vi "NMLDAQ_data_import.vi"(0 "NML Data Acquisition VI":string(combo)="NML Data Acquisition-New.vi") -> (1 "data":dbl[][](array[numeric])=[[0.0, 0.0], [0.481, 0.481], [0.98, 0.98], [1.48, 1.48], [1.98, 1.98], [2.48, 2.48], [2.98, 2.98], [3.48, 3.48], [3.98, 3.98], [4.48, 4.48], [4.98, 4.98], [5.48, 5.48], [5.98, 5.98], [6.48, 6.48], [6.98, 6.98], [7.48, 7.48], [7.98, 7.98], [8.48, 8.48], [8.98, 8.98], [9.48, 9.48], [9.98, 9.98], [10.48, 10.48], [10.98, 10.98], [11.48, 11.48], [11.981, 11.981], [12.48, 12.48], [12.981, 12.981], [13.48, 13.48], [13.98, 13.98], [14.48, 14.48], [14.98, 14.98], [15.48, 15.48], [15.981, 15.981], [16.48, 16.48], [16.981, 16.981], [17.48, 17.48], [17.98, 17.98], [18.48, 18.48], [18.981, 18.981], [19.48, 19.48], [19.98, 19.98], [20.48, 20.48], [20.981, 20.981], [21.48, 21.48], [21.981, 21.981], [22.48, 22.48], [22.981, 22.981], [23.48, 23.48], [23.981, 23.981], [24.48, 24.48], [24.981, 24.981], [25.48, 25.48], [25.98, 25.98], [26.48, 26.48], [26.981, 26.981], [27.48, 27.48], [27.981, 27.981], [28.48, 28.48], [28.981, 28.981], [29.48, 29.48], [29.981, 29.981], [30.48, 30.48], [30.981, 30.981], [31.48, 31.48], [31.98, 31.98], [32.48, 32.48], [32.98, 32.98], [33.48, 33.48], [33.98, 33.98], [34.48, 34.48], [34.98, 34.98], [35.48, 35.48], [35.98, 35.98], [36.48, 36.48], [36.98, 36.98], [37.48, 37.48], [37.98, 37.98], [38.48, 38.48], [38.98, 38.98], [39.48, 39.48], [39.98, 39.98], [40.48, 40.48], [40.98, 40.98], [41.48, 41.48], [41.98, 41.98], [42.48, 42.48], [42.98, 42.98], [43.48, 43.48], [43.98, 43.98], [44.48, 44.48], [44.98, 44.98], [45.48, 45.48], [45.98, 45.98], [46.481, 46.481], [46.98, 46.98], [47.48, 47.48], [47.98, 47.98], [48.48, 48.48], [48.98, 48.98], [49.48, 49.48], [49.98, 49.98], [50.48, 50.48], [50.98, 50.98], [51.48, 51.48], [51.981, 51.981], [52.48, 52.48], [52.981, 52.981], [53.48, 53.48], [53.981, 53.981], [54.48, 54.48], [54.981, 54.981], [55.48, 55.48], [55.981, 55.981], [56.481, 56.481], [56.98, 56.98], [57.48, 57.48], [57.98, 57.98], [58.48, 58.48], [58.98, 58.98], [59.48, 59.48], [59.98, 59.98], [60.48, 60.48], [60.98, 60.98], [61.48, 61.48], [61.98, 61.98], [62.48, 62.48], [62.98, 62.98], [63.48, 63.48], [63.98, 63.98], [64.48, 64.48], [64.98, 64.98], [65.48, 65.48], [65.98, 65.98], [66.481, 66.481], [66.98, 66.98], [67.48, 67.48], [67.98, 67.98], [68.48, 68.48], [68.98, 68.98], [69.48, 69.48], [69.98, 69.98], [70.48, 70.48], [70.98, 70.98], [71.48, 71.48], [71.981, 71.981], [72.48, 72.48], [72.98, 72.98], [73.48, 73.48], [73.98, 73.98], [74.48, 74.48], [74.98, 74.98], [75.48, 75.48], [75.98, 75.98], [76.48, 76.48], [76.98, 76.98], [77.48, 77.48], [77.981, 77.981], [78.48, 78.48], [78.981, 78.981], [79.48, 79.48], [79.981, 79.981], [80.48, 80.48], [80.981, 80.981], [81.48, 81.48], [81.981, 81.981], [82.48, 82.48], [82.981, 82.981], [83.48, 83.48], [83.981, 83.981], [84.48, 84.48], [84.981, 84.981], [85.48, 85.48], [85.981, 85.981], [86.48, 86.48], [86.98, 86.98], [87.48, 87.48], [87.981, 87.981], [88.48, 88.48], [88.981, 88.981], [89.48, 89.48], [89.98, 89.98], [90.48, 90.48], [90.98, 90.98], [91.48, 91.48], [91.98, 91.98], [92.48, 92.48], [92.98, 92.98], [93.48, 93.48], [93.98, 93.98], [94.48, 94.48], [94.98, 94.98], [95.48, 95.48], [95.981, 95.981], [96.48, 96.48], [96.98, 96.98], [97.48, 97.48], [97.98, 97.98], [98.48, 98.48], [98.981, 98.981], [99.48, 99.48], [99.981, 99.981], [100.48, 100.48], [100.98, 100.98], [101.48, 101.48], [101.981, 101.981], [102.48, 102.48], [102.981, 102.981], [103.48, 103.48], [103.981, 103.981], [104.48, 104.48], [104.98, 104.98], [105.48, 105.48], [105.98, 105.98], [106.48, 106.48], [106.981, 106.981], [107.48, 107.48], [107.981, 107.981], [108.48, 108.48], [108.981, 108.981], [109.48, 109.48], [109.981, 109.981], [110.48, 110.48], [110.981, 110.981], [111.48, 111.48], [111.981, 111.981], [112.48, 112.48], [112.981, 112.981], [113.48, 113.48], [113.981, 113.981], [114.48, 114.48], [114.981, 114.981], [115.48, 115.48], [115.981, 115.981], [116.48, 116.48], [116.981, 116.981], [117.48, 117.48], [117.981, 117.981], [118.48, 118.48], [118.981, 118.981], [119.48, 119.48], [119.981, 119.981], [120.48, 120.48], [120.981, 120.981], [121.48, 121.48], [121.981, 121.981], [122.48, 122.48], [122.981, 122.981], [123.48, 123.48], [123.981, 123.981], [124.48, 124.48], [124.981, 124.981], [125.48, 125.48], [125.981, 125.981], [126.48, 126.48], [126.981, 126.981], [127.48, 127.48], [127.981, 127.981], [128.48, 128.48], [128.981, 128.981], [129.48, 129.48], [129.981, 129.981], [130.48, 130.48], [130.981, 130.981], [131.48, 131.48], [131.981, 131.981], [132.48, 132.48], [132.981, 132.981], [133.48, 133.48], [133.981, 133.981], [134.48, 134.48], [134.981, 134.981], [135.48, 135.48], [135.981, 135.981], [136.48, 136.48], [136.981, 136.981], [137.48, 137.48], [137.981, 137.981], [138.48, 138.48], [138.981, 138.981], [139.48, 139.48], [139.981, 139.981], [140.48, 140.48], [140.981, 140.981], [141.48, 141.48], [141.981, 141.981], [142.48, 142.48], [142.981, 142.981], [143.48, 143.48], [143.981, 143.981], [144.48, 144.48], [144.981, 144.981], [145.48, 145.48], [145.981, 145.981], [146.48, 146.48], [146.981, 146.981], [147.48, 147.48], [147.981, 147.981], [148.48, 148.48], [148.981, 148.981], [149.48, 149.48], [149.981, 149.981], [150.48, 150.48], [150.981, 150.981], [151.48, 151.48], [151.981, 151.981], [152.48, 152.48], [152.98, 152.98], [153.48, 153.48], [153.981, 153.981], [154.48, 154.48], [154.981, 154.981], [155.48, 155.48], [155.981, 155.981], [156.48, 156.48], [156.981, 156.981], [157.48, 157.48], [157.98, 157.98], [158.48, 158.48], [158.981, 158.981], [159.48, 159.48], [159.98, 159.98], [160.48, 160.48], [160.981, 160.981], [161.48, 161.48], [161.981, 161.981], [162.48, 162.48], [162.98, 162.98], [163.48, 163.48], [163.98, 163.98], [164.48, 164.48], [164.98, 164.98], [165.48, 165.48], [165.981, 165.981], [166.48, 166.48], [166.981, 166.981], [167.48, 167.48], [167.981, 167.981], [168.48, 168.48], [168.98, 168.98], [169.48, 169.48], [169.981, 169.981], [170.48, 170.48], [170.981, 170.981], [171.48, 171.48], [171.981, 171.981], [172.48, 172.48], [172.98, 172.98], [173.48, 173.48], [173.98, 173.98], [174.48, 174.48], [174.981, 174.981], [175.48, 175.48], [nan, nan], [nan, nan], [nan, nan], [nan, nan], [nan, nan], [nan, nan], [nan, nan], [nan, nan], [nan, nan], [nan, nan], [nan, nan], [nan, nan], [nan, nan], [nan, nan], [nan, nan], [nan, nan], [nan, nan], [nan, nan], [nan, nan], [nan, nan], [nan, nan], [nan, nan], [nan, nan], [nan, nan], [nan, nan], [nan, nan], [nan, nan], [nan, nan], [nan, nan], [nan, nan], [nan, nan], [nan, nan], [nan, nan], [nan, nan], [nan, nan], [nan, nan], [nan, nan], [nan, nan], [nan, nan], [nan, nan], [nan, nan], [nan, nan], [nan, nan], [nan, nan], [nan, nan], [nan, nan], [nan, nan], [nan, nan], [nan, nan], [nan, nan], [nan, nan], [nan, nan], [nan, nan], [nan, nan], [nan, nan], [nan, nan], [nan, nan], [nan, nan], [nan, nan], [nan, nan], [nan, nan], [nan, nan], [nan, nan], [nan, nan], [nan, nan], [nan, nan], [nan, nan], [nan, nan], [nan, nan], [nan, nan], [nan, nan], [nan, nan], [nan, nan], [nan, nan], [nan, nan], [nan, nan], [nan, nan], [nan, nan], [nan, nan], [nan, nan], [nan, nan], [nan, nan], [nan, nan], [nan, nan], [nan, nan], [nan, nan], [nan, nan], [nan, nan], [nan, nan], [nan, nan], [nan, nan], [nan, nan], [nan, nan], [nan, nan], [nan, nan], [nan, nan], [nan, nan], [nan, nan], [nan, nan], [nan, nan], [nan, nan], [nan, nan], [nan, nan], [nan, nan], [nan, nan], [nan, nan], [nan, nan], [nan, nan], [nan, nan], [nan, nan], [nan, nan], [nan, nan], [nan, nan], [nan, nan], [nan, nan], [nan, nan], [nan, nan], [nan, nan], [nan, nan], [nan, nan], [nan, nan], [nan, nan], [nan, nan], [nan, nan], [nan, nan], [nan, nan], [nan, nan], [nan, nan], [nan, nan], [nan, nan], [nan, nan], [nan, nan], [nan, nan], [nan, nan], [nan, nan], [nan, nan], [nan, nan], [nan, nan], [nan, nan], [nan, nan], [nan, nan], [nan, nan], [nan, nan], [nan, nan], [nan, nan], [nan, nan], [nan, nan], [nan, nan], [nan, nan], [nan, nan], [nan, nan], [nan, nan], [nan, nan], [nan, nan], [nan, nan], [nan, nan], [nan, nan], [nan, nan], [nan, nan], [nan, nan], [nan, nan], [nan, nan], [nan, nan], [nan, nan], [nan, nan], [nan, nan], [nan, nan], [nan, nan], [nan, nan], [nan, nan], [nan, nan], [nan, nan], [nan, nan], [nan, nan], [nan, nan], [nan, nan], [nan, nan], [nan, nan], [nan, nan], [nan, nan], [nan, nan], [nan, nan], [nan, nan], [nan, nan], [nan, nan], [nan, nan], [nan, nan], [nan, nan], [nan, nan], [nan, nan], [nan, nan], [nan, nan], [nan, nan], [nan, nan], [nan, nan], [nan, nan], [nan, nan], [nan, nan], [nan, nan], [nan, nan], [nan, nan], [nan, nan], [nan, nan], [nan, nan], [nan, nan], [nan, nan], [nan, nan], [nan, nan], [nan, nan], [nan, nan], [nan, nan], [nan, nan], [nan, nan], [nan, nan], [nan, nan], [nan, nan], [nan, nan], [nan, nan], [nan, nan], [nan, nan], [nan, nan], [nan, nan], [nan, nan], [nan, nan], [nan, nan], [nan, nan], [nan, nan], [nan, nan], [nan, nan], [nan, nan], [nan, nan], [nan, nan], [nan, nan], [nan, nan], [nan, nan], [nan, nan], [nan, nan], [nan, nan], [nan, nan], [nan, nan], [nan, nan], [nan, nan], [nan, nan], [nan, nan], [nan, nan], [nan, nan], [nan, nan], [nan, nan], [nan, nan], [nan, nan], [nan, nan], [nan, nan], [nan, nan], [nan, nan], [nan, nan], [nan, nan], [nan, nan], [nan, nan], [nan, nan], [nan, nan], [nan, nan], [nan, nan], [nan, nan], [nan, nan], [nan, nan], [nan, nan], [nan, nan], [nan, nan], [nan, nan], [nan, nan], [nan, nan], [nan, nan], [nan, nan], [nan, nan], [nan, nan], [nan, nan], [nan, nan], [nan, nan], [nan, nan], [nan, nan], [nan, nan], [nan, nan], [nan, nan], [nan, nan], [nan, nan], [nan, nan], [nan, nan], [nan, nan], [nan, nan], [nan, nan], [nan, nan], [nan, nan], [nan, nan], [nan, nan], [nan, nan], [nan, nan], [nan, nan], [nan, nan], [nan, nan], [nan, nan], [nan, nan], [nan, nan], [nan, nan], [nan, nan], [nan, nan], [nan, nan], [nan, nan], [nan, nan], [nan, nan], [nan, nan], [nan, nan], [nan, nan], [nan, nan], [nan, nan], [nan, nan], [nan, nan], [nan, nan], [nan, nan], [nan, nan], [nan, nan], [nan, nan], [nan, nan], [nan, nan], [nan, nan], [nan, nan], [nan, nan], [nan, nan], [nan, nan], [nan, nan], [nan, nan], [nan, nan], [nan, nan], [nan, nan], [nan, nan], [nan, nan], [nan, nan], [nan, nan], [nan, nan], [nan, nan], [nan, nan], [nan, nan], [nan, nan], [nan, nan], [nan, nan], [nan, nan], [nan, nan], [nan, nan], [nan, nan], [nan, nan], [nan, nan], [nan, nan], [nan, nan], [nan, nan], [nan, nan], [nan, nan], [nan, nan], [nan, nan], [nan, nan], [nan, nan], [nan, nan], [nan, nan], [nan, nan], [nan, nan], [nan, nan], [nan, nan], [nan, nan], [nan, nan], [nan, nan], [nan, nan], [nan, nan], [nan, nan], [nan, nan], [nan, nan], [nan, nan], [nan, nan], [nan, nan], [nan, nan], [nan, nan], [nan, nan], [nan, nan], [nan, nan], [nan, nan], [nan, nan], [nan, nan], [nan, nan], [nan, nan], [nan, nan], [nan, nan], [nan, nan], [nan, nan], [nan, nan], [nan, nan], [nan, nan], [nan, nan], [nan, nan], [nan, nan], [nan, nan], [nan, nan], [nan, nan], [nan, nan], [nan, nan], [nan, nan], [nan, nan], [nan, nan], [nan, nan], [nan, nan], [nan, nan], [nan, nan], [nan, nan], [nan, nan], [nan, nan], [nan, nan], [nan, nan], [nan, nan], [nan, nan], [nan, nan], [nan, nan], [nan, nan], [nan, nan], [nan, nan], [nan, nan], [nan, nan], [nan, nan], [nan, nan], [nan, nan], [nan, nan], [nan, nan], [nan, nan], [nan, nan], [nan, nan], [nan, nan], [nan, nan], [nan, nan], [nan, nan], [nan, nan], [nan, nan], [nan, nan], [nan, nan], [nan, nan], [nan, nan], [nan, nan], [nan, nan], [nan, nan], [nan, nan], [nan, nan], [nan, nan], [nan, nan], [nan, nan], [nan, nan], [nan, nan], [nan, nan], [nan, nan], [nan, nan], [nan, nan], [nan, nan], [nan, nan], [nan, nan], [nan, nan], [nan, nan], [nan, nan], [nan, nan], [nan, nan], [nan, nan], [nan, nan], [nan, nan], [nan, nan], [nan, nan], [nan, nan], [nan, nan], [nan, nan], [nan, nan], [nan, nan], [nan, nan], [nan, nan], [nan, nan], [nan, nan], [nan, nan], [nan, nan], [nan, nan], [nan, nan], [nan, nan], [nan, nan], [nan, nan], [nan, nan], [nan, nan], [nan, nan], [nan, nan], [nan, nan], [nan, nan], [nan, nan], [nan, nan], [nan, nan], [nan, nan], [nan, nan], [nan, nan], [nan, nan], [nan, nan], [nan, nan], [nan, nan], [nan, nan], [nan, nan], [nan, nan], [nan, nan], [nan, nan], [nan, nan], [nan, nan], [nan, nan], [nan, nan], [nan, nan], [nan, nan], [nan, nan], [nan, nan], [nan, nan], [nan, nan], [nan, nan], [nan, nan], [nan, nan], [nan, nan], [nan, nan], [nan, nan], [nan, nan], [nan, nan], [nan, nan], [nan, nan], [nan, nan], [nan, nan], [nan, nan], [nan, nan], [nan, nan], [nan, nan], [nan, nan], [nan, nan], [nan, nan], [nan, nan], [nan, nan], [nan, nan], [nan, nan], [nan, nan], [nan, nan], [nan, nan], [nan, nan], [nan, nan], [nan, nan], [nan, nan], [nan, nan], [nan, nan], [nan, nan], [nan, nan], [nan, nan], [nan, nan], [nan, nan], [nan, nan], [nan, nan], [nan, nan], [nan, nan], [nan, nan], [nan, nan], [nan, nan], [nan, nan], [nan, nan], [nan, nan], [nan, nan], [nan, nan], [nan, nan], [nan, nan], [nan, nan], [nan, nan], [nan, nan], [nan, nan], [nan, nan], [nan, nan], [nan, nan], [nan, nan], [nan, nan], [nan, nan], [nan, nan], [nan, nan], [nan, nan], [nan, nan], [nan, nan], [nan, nan], [nan, nan], [nan, nan], [nan, nan], [nan, nan], [nan, nan], [nan, nan], [nan, nan], [nan, nan], [nan, nan], [nan, nan], [nan, nan], [nan, nan], [nan, nan], [nan, nan], [nan, nan], [nan, nan], [nan, nan], [nan, nan], [nan, nan], [nan, nan], [nan, nan], [nan, nan], [nan, nan], [nan, nan], [nan, nan], [nan, nan], [nan, nan], [nan, nan], [nan, nan], [nan, nan], [nan, nan], [nan, nan], [nan, nan], [nan, nan], [nan, nan], [nan, nan], [nan, nan], [nan, nan], [nan, nan], [nan, nan], [nan, nan], [nan, nan], [nan, nan], [nan, nan], [nan, nan], [nan, nan], [nan, nan], [nan, nan], [nan, nan], [nan, nan], [nan, nan], [nan, nan], [nan, nan], [nan, nan], [nan, nan], [nan, nan], [nan, nan], [nan, nan], [nan, nan], [nan, nan], [nan, nan], [nan, nan], [nan, nan], [nan, nan], [nan, nan], [nan, nan], [nan, nan], [nan, nan], [nan, nan], [nan, nan], [nan, nan], [nan, nan], [nan, nan], [nan, nan], [nan, nan], [nan, nan], [nan, nan], [nan, nan], [nan, nan], [nan, nan], [nan, nan], [nan, nan], [nan, nan], [nan, nan], [nan, nan], [nan, nan], [nan, nan], [nan, nan], [nan, nan], [nan, nan], [nan, nan]], 2 "file name":string, 3 "error out":errorcluster)   [LabVIEW 2021]
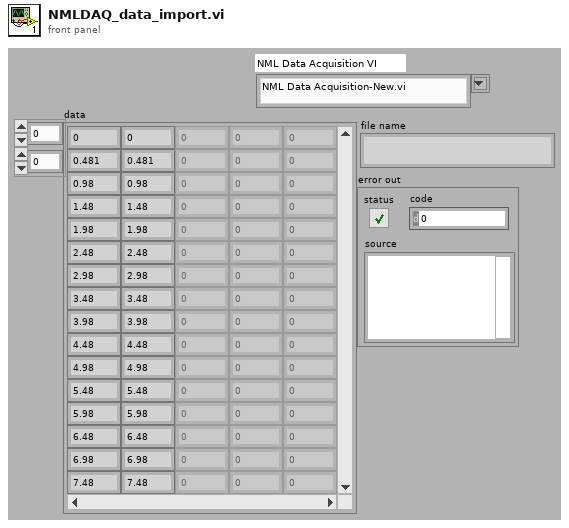
[diagram p1: front panel]
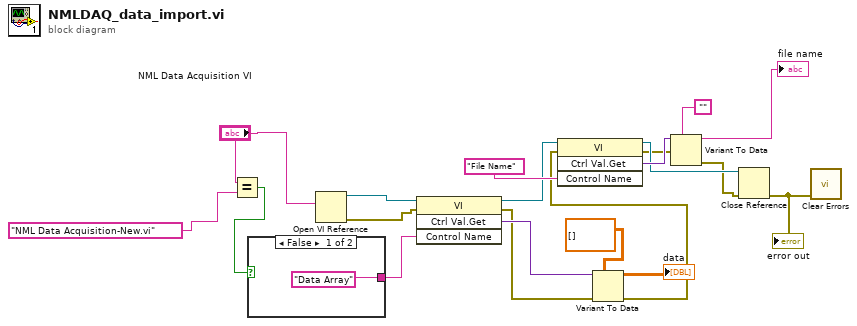
[diagram p0: block diagram]
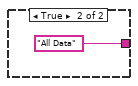
[diagram p2: hidden frame]
diagram:
  n1 = Equal?(x="NML Data Acquisition VI", y="NML Data Acquisition-New.vi" ("NML Data Acquisition VI")) -> (x = y?=w14:bool)
  n2 = case shown="False" w14 {
    tunnel: ["Data Array" ("Control Name") "All Data" ("Control Name")] -> w16
    frame False {
    }
    frame True {
    }
  }
  n3 = Open VI Reference(vi path="NML Data Acquisition VI") -> (vi reference=w9:refnum<vi>, error out=w18:errorcluster)  [unwired: 1 in, 4 out]
  n4 = invoke class="VI" method="Ctrl Val.Get"(reference=w9, error in=w18, "Control Name"=w16) -> (reference out=w8:refnum<vi>, error out=w2:errorcluster, "Get Control Value Variant"=w17:variant)  [unwired: 1 in, 1 out]
  n5 = Variant To Data(error in=w2, type=dbl[][] [] ("data"), Variant=w17) -> (data=→"data":dbl[][], error out=w1:errorcluster)
  n6 = invoke class="VI" method="Ctrl Val.Get"(reference=w8, error in=w1, "Control Name"="File Name") -> (reference out=w7:refnum<vi>, error out=w5:errorcluster, "Get Control Value Variant"=w12:variant)  [unwired: 1 in, 1 out]
  n7 = Variant To Data(error in=w5, type="", Variant=w12) -> (data=→"file name":string, error out=w4:errorcluster)
  n8 = Close Reference(reference=w7, error in (no error)=w4) -> (error out=w3:errorcluster)
  "error out" <- w3
  n9 = call <vilib>:"Clear Errors.vi"("error in (no error)"=w3) -> ()  [unwired: 5 in, 2 out]
